vi "GraphSetting Get PlotName (Wave).vi"(8 "error in (no error)":errorcluster caption="エラー入力（エラーなし）", 11 "波形グラフref(in)":refnum<vi>) -> (0 "error out":errorcluster caption="エラー出力", 2 "プロット名称[]":string[](array[string]))   [LabVIEW 2014]
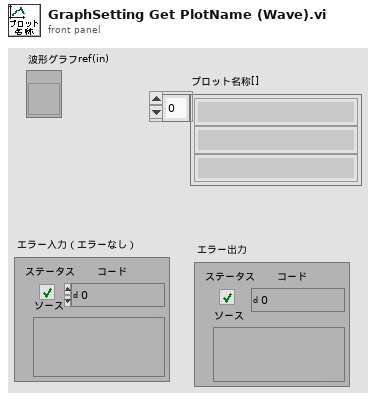
[diagram p1: front panel]
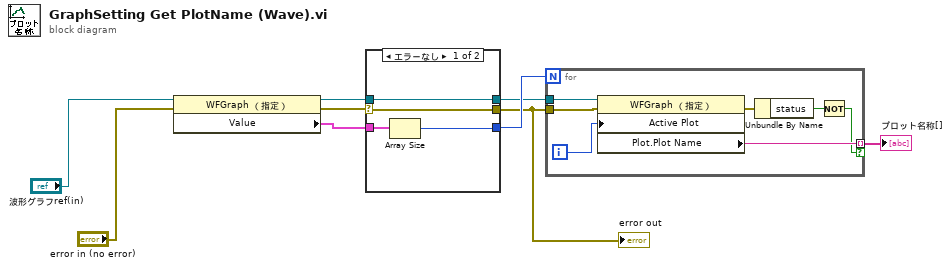
[diagram p0: block diagram]
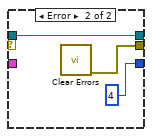
[diagram p2: hidden frame]
diagram:
  n1 = property class="WFGraph （指定）"(reference="波形グラフref(in)", error in="error in (no error)") -> (reference out=w2:refnum<vi>, error out=w4:errorcluster, "Value"=w8:cluster{dbl, "dt":dbl, "Y":dbl[]}[])
  n2 = case shown="エラーなし" w4 {
    selector: w4 -> [w10 _]
    tunnel: w8 -> [w13 _]
    tunnel: [w12 4] -> w5
    tunnel: [w10 w16] -> w1
    tunnel: [w11 w15] -> w3
    tunnel: w2 -> [w11 w15]
    frame No Error {
      n3 = Array Size(array=w13) -> (size(s)=w12:i32)
    }
    frame Error {
      n4 = call <vilib>:"Clear Errors.vi"() -> ("error out"=w16:errorcluster)  [unwired: 6 in, 1 out]
    }
  }
  "error out" <- w1
  n5 = for {
    N: w5 -> [_]
    tunnel: w3 -> [w23]
    tunnel: [w22] -> w9 mode=indexing if=w19
    tunnel: w1 -> [w18]
    i -> [w17]
    n6 = property class="WFGraph （指定）"(reference=w23, error in=w18, "Active Plot"=w17) -> (error out=w21:errorcluster, "Plot.Plot Name"=w22:string)  [unwired: 1 out]
    n7 = Unbundle By Name(w21) -> ("status"=w20:bool)
    n8 = Not(x=w20) -> (.not. x?=w19:bool)
  }
  "プロット名称[]" <- w9
